vi "cintaindexada.vi"() -> ()   [LabVIEW 2017]
panel:
  out "Numeric":dbl
  out "Boolean 2":bool
  in  "reset":bool
  in  "stop":bool
  in  "Boolean":bool
  out "Slide":dbl(slide) scale=0.0..10.0
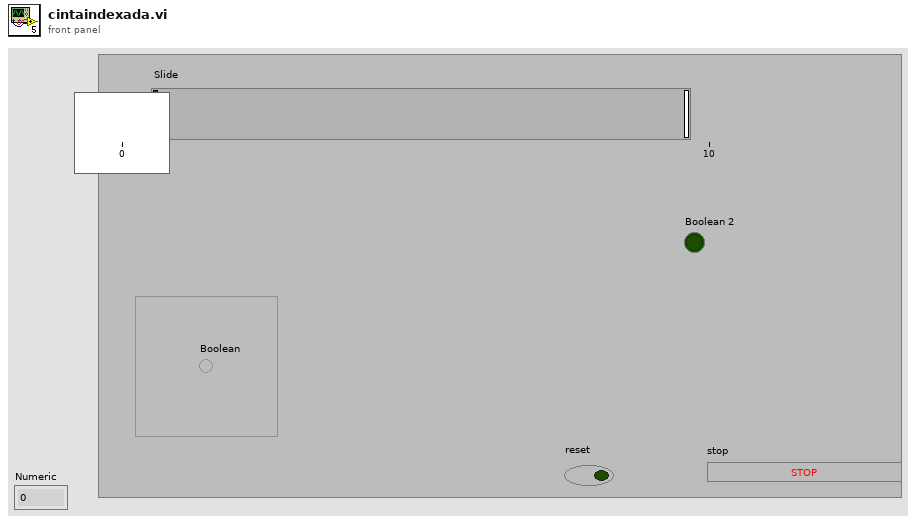
[diagram p1: front panel]
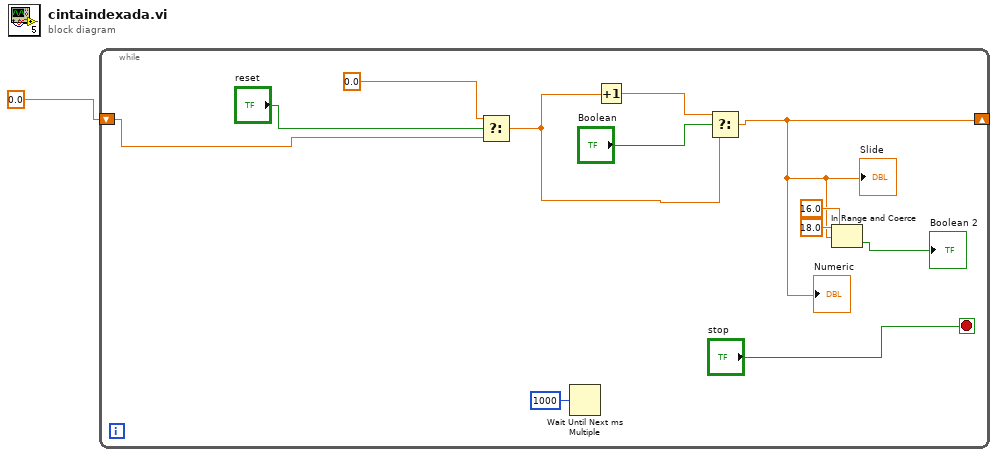
[diagram p0: block diagram]
diagram:
  n1 = while {
    shift-right: [w2] -> _
    shift-left: 0.0 -> [w11]
    stop <- "stop" stop-if-true
    n2 = Select(t=0.0, s="reset", f=w11) -> (s? t:f=w7:dbl)
    n3 = Wait Until Next ms Multiple(millisecond multiple=u32 1000) -> ()  [unwired: 1 out]
    n4 = Increment(x=w7) -> (x+1=w10:dbl)
    n5 = Select(t=w10, s="Boolean", f=w7) -> (s? t:f=w2:dbl)
    "Slide" <- w2
    "Numeric" <- w2
    n6 = In Range and Coerce(upper limit=18.0, x=w2, lower limit=16.0) -> (In Range?=→"Boolean 2":bool)  [unwired: 1 out]
  }
